vi "Insert.vi"(1 "Count":i32=2000) -> (0 "Inser String":string)   [LabVIEW 2020]
uses:
  <vilib>/measure/NI_MABase.lvlib
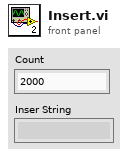
[diagram p1: front panel]
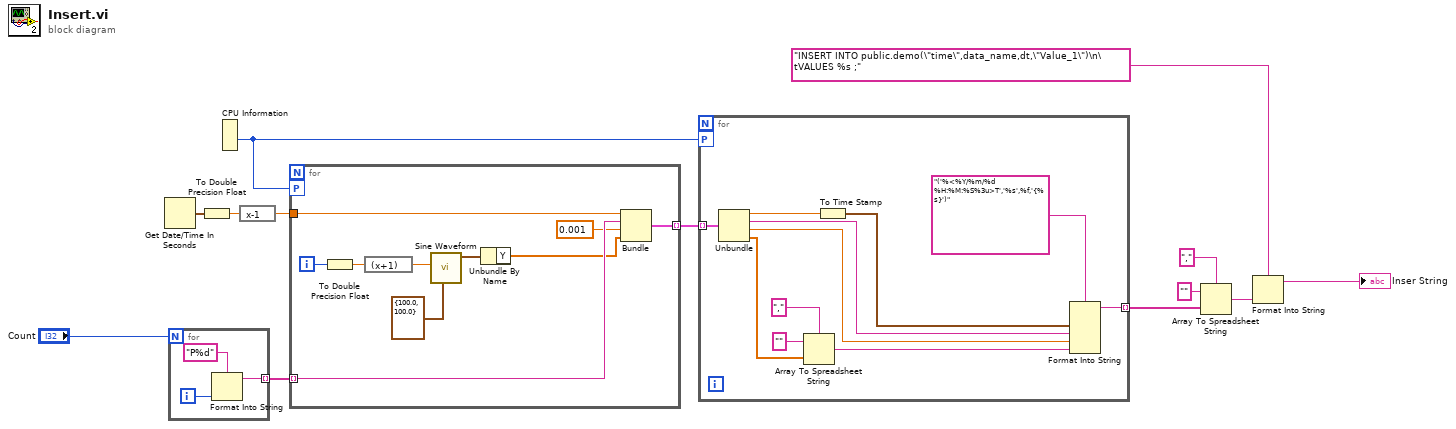
[diagram p0: block diagram]
diagram:
  n1 = Get Date/Time In Seconds() -> (seconds since 1Jan1904=w10:timestamp)
  n2 = for {
    N: "Count" -> [_]
    tunnel: [w14] -> w11 mode=indexing
    i -> [w16]
    n3 = Format Into String(format string="P%d", w16) -> (resulting string=w14:string)  [unwired: 2 in, 1 out]
  }
  n4 = To Double Precision Float(number=w10) -> (double precision float=w3:dbl)
  n5 = CPU Information() -> (6:w1:i32)  [unwired: 3 out]
  n6 = expression code="x-1"(w3) -> (w2:dbl)
  n7 = for {
    tunnel: w11 -> [w26] mode=indexing
    tunnel: w2 -> [w23]
    workers-P: w1 -> [_]
    tunnel: [w24] -> w4 mode=indexing
    i -> [w21]
    n8 = To Double Precision Float(number=w21) -> (double precision float=w19:dbl)
    n9 = expression code="(x+1)"(w19) -> (w18:dbl)
    n10 = call <vilib>:"Sine Waveform.vi"("sampling info"=cluster{"Fs":dbl, "#s":dbl} {"Fs"=100.0, "#s"=100.0}, "amplitude"=w18) -> ("signal out"=w20:waveform(dbl))  [unwired: 8 in, 1 out]
    n11 = Unbundle By Name(w20) -> ("Y"=w17:dbl[])
    n12 = Bundle(w23, w26, 0.001, "Y"=w17) -> (w24:cluster{dbl, string, dbl, "Y":dbl[]})  [unwired: 1 in]
  }
  n13 = for {
    tunnel: [w35] -> w9 mode=indexing
    workers-P: w1 -> [_]
    tunnel: w4 -> [w31] mode=indexing
    n14 = Unbundle(w31) -> (w34:dbl, w33:string, w32:dbl, "Y"=w28:dbl[])
    n15 = Array To Spreadsheet String(delimiter (Tab)=",", array=w28, 3:"" ("format string")) -> (spreadsheet string=w27:string)
    n16 = To Time Stamp(1:w34) -> (0:w37:timestamp)
    n17 = Format Into String(format string="('%<%Y/%m/%d %H:%M:%S%3u>T','%s',%f,'{%s}')", w37, w33, w32, w27) -> (resulting string=w35:string)  [unwired: 2 in, 1 out]
  }
  n18 = Array To Spreadsheet String(delimiter (Tab)=",", array=w9, 3:"" ("format string")) -> (spreadsheet string=w6:string)
  n19 = Format Into String(format string="INSERT INTO public.demo(\"time\",data_name,dt,\"Value_1\")\n\tVALUES %s ;", w6) -> (resulting string=→"Inser String":string)  [unwired: 2 in, 1 out]
